vi "init daq state.vi"(0 "Default Setpoint (C)":dbl=30.0, 7 "DAQ state start in":T8 {"T cont"."utility"."therm volt" format="%_6g"; "T cont"."utility"."heat volt in" format="%_6g"; "T cont"."utility"."heat volt out" format="%_6g"; "T cont"."utility"."power out" format="%_6g"; "T cont"."utility"."H Vmax" format="%_6g"; "T cont"."exec"."man power" format="%_6g"; "T cont"."exec"."exec setpoint" format="%_6g"; "T cont"."T params"."Settle Time" step=1.0; "T cont"."T params"."Settle Bandwidth" step=0.01; "T cont"."T params"."Derivative Tme" step=0.01; "T cont"."T params"."Integral Time" step=1.0; "T cont"."T params"."Control Bandwidth" step=0.1; "T cont"."T params"."Setpoint" step=0.1; "T cont"."T status"."Setpoint" format="%_6g"; "T cont"."T status"."Power" format="%_6g"; "T cont"."T status"."Temp" format="%_6g"}, 11 "T cont wait time (ms)":i32=300) -> (4 "T cont out for global update":T1={"exec"={"T mode"=enum."Listening to exec", "exec setpoint"=30.0, "reset"=FALSE, "man power"=0.5, "man"=FALSE, "log"=FALSE, "clear"=FALSE}, "T status"={"Control status"=enum."Below Control Band", "Temp"=0.0, "Power"=0.0, "Time in settle band"=0.0, "Settled"=FALSE, "Low"=FALSE, "High"=FALSE, "Setpoint"=30.0, "Control"=FALSE, "In Settle Band"=FALSE}, "T params"={"Setpoint"=30.0, "Control Bandwidth"=4.0, "Integral Time"=30.0, "Int\nON"=TRUE, "Derivative Tme"=0.5, "Der\nON"=TRUE, "Settle Bandwidth"=1.0, "Settle Time"=60.0}, "utility"={"meas index"=0, "wait (ms)"=300, "H Vmax"=8.5, "power out"=0.0, "heat volt out"=0.0, "heat volt in"=0.0, "therm volt"=0.0, "t T P hist"=[], "cont hist"=[]}} {"utility"."therm volt" format="%_6g"; "utility"."heat volt in" format="%_6g"; "utility"."heat volt out" format="%_6g"; "utility"."power out" format="%_6g"; "utility"."H Vmax" format="%_6g"; "exec"."man power" format="%_6g"; "exec"."exec setpoint" format="%_6g"; "T params"."Settle Time" step=1.0; "T params"."Settle Bandwidth" step=0.01; "T params"."Derivative Tme" step=0.01; "T params"."Integral Time" step=1.0; "T params"."Control Bandwidth" step=0.1; "T params"."Setpoint" step=0.1; "T status"."Setpoint" format="%_6g"; "T status"."Power" format="%_6g"; "T status"."Temp" format="%_6g"}, 8 "DAQ state start out":T8 {"T cont"."utility"."therm volt" format="%_6g"; "T cont"."utility"."heat volt in" format="%_6g"; "T cont"."utility"."heat volt out" format="%_6g"; "T cont"."utility"."power out" format="%_6g"; "T cont"."utility"."H Vmax" format="%_6g"; "T cont"."exec"."man power" format="%_6g"; "T cont"."exec"."exec setpoint" format="%_6g"; "T cont"."T params"."Settle Time" step=1.0; "T cont"."T params"."Settle Bandwidth" step=0.01; "T cont"."T params"."Derivative Tme" step=0.01; "T cont"."T params"."Integral Time" step=1.0; "T cont"."T params"."Control Bandwidth" step=0.1; "T cont"."T params"."Setpoint" step=0.1; "T cont"."T status"."Setpoint" format="%_6g"; "T cont"."T status"."Power" format="%_6g"; "T cont"."T status"."Temp" format="%_6g"})   [LabVIEW 2019]
doc: "Thus subvi initializes the temp daq state machine and the global variables for the bug experiment.\n\nPaul K Dixon\nP3600\nCSUSB Physics"
uses:
  typedefs/DAQ T state cluster.ctl
  typedefs/DAQ T state enum.ctl
  typedefs/temp cont cluster.ctl
  typedefs/temp exec cluster.ctl
  typedefs/temp mode enum.ctl
  typedefs/temp indicator.ctl
  typedefs/temp control status.ctl
  typedefs/PID control parameters.ctl
  typedefs/temp cont utility.ctl
panel:
  in  "T cont.T status":T4={"Control status"=enum."Below Control Band", "Temp"=25.0, "Power"=0.0, "Time in settle band"=0.0, "Settled"=FALSE, "Low"=TRUE, "High"=FALSE, "Setpoint"=30.0, "Control"=FALSE, "In Settle Band"=FALSE} {"Setpoint" format="%_6g"; "Power" format="%_6g"; "Temp" format="%_6g"}
  in  "T cont.T params":T6={"Setpoint"=30.0, "Control Bandwidth"=4.0, "Integral Time"=20.0, "Int\nON"=TRUE, "Derivative Tme"=0.2, "Der\nON"=TRUE, "Settle Bandwidth"=1.0, "Settle Time"=60.0} {"Settle Time" step=1.0; "Settle Bandwidth" step=0.01; "Derivative Tme" step=0.01; "Integral Time" step=1.0; "Control Bandwidth" step=0.1; "Setpoint" step=0.1}
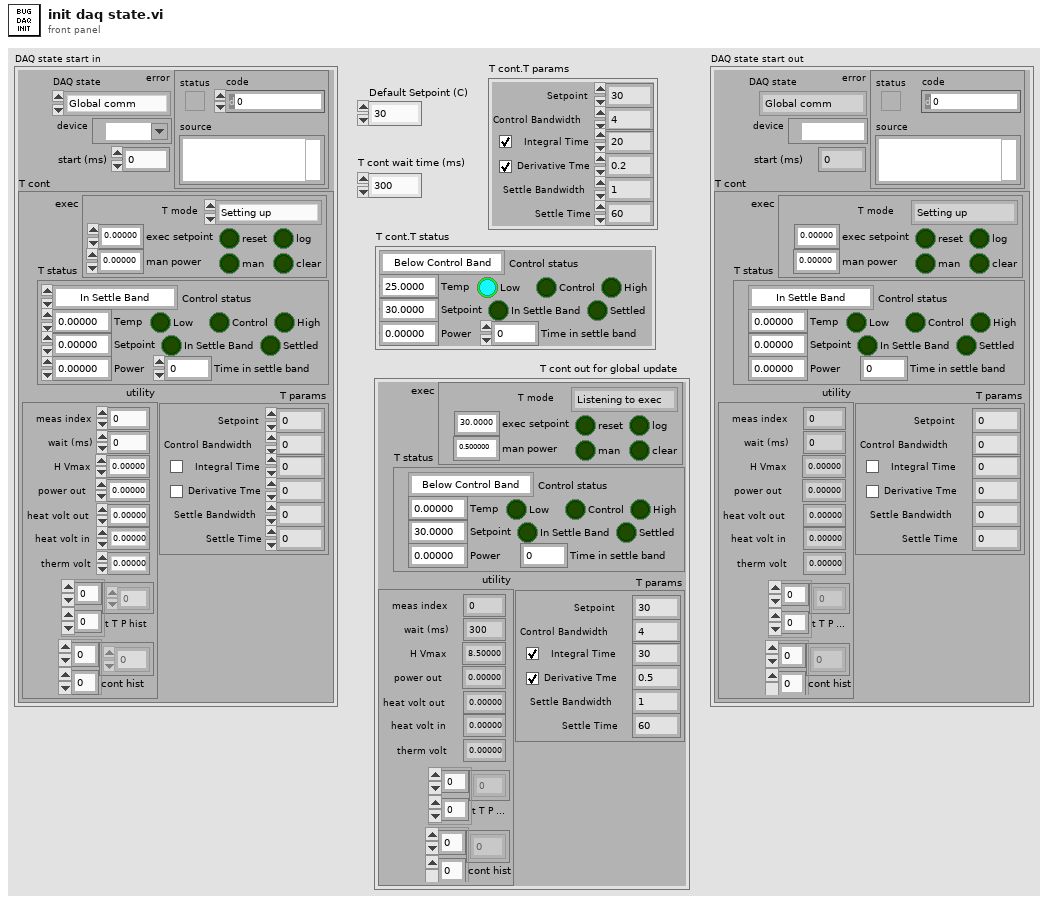
[diagram p1: front panel]
types:
  T1 = typedef "temp cont cluster.ctl" = cluster{"exec":T2, "T status":T4, "T params":T6, "utility":T7}
  T2 = typedef "temp exec cluster.ctl" = cluster{"T mode":T3, "exec setpoint":dbl, "reset":bool, "man power":dbl, "man":bool, "log":bool, "clear":bool}
  T3 = typedef "temp mode enum.ctl" = enum16{"Setting up", "Listening to exec", "Exit"}
  T4 = typedef "temp indicator.ctl" = cluster{"Control status":T5, "Temp":dbl, "Power":dbl, "Time in settle band":dbl, "Settled":bool, "Low":bool, "High":bool, "Setpoint":dbl, "Control":bool, "In Settle Band":bool}
  T5 = typedef "temp control status.ctl" = enum16{"In Settle Band", "In Control Band", "Below Control Band", "Above Control Band"}
  T6 = typedef "PID control parameters.ctl" = cluster{"Setpoint":dbl, "Control Bandwidth":dbl, "Integral Time":dbl, "Int\nON":bool, "Derivative Tme":dbl, "Der\nON":bool, "Settle Bandwidth":dbl, "Settle Time":dbl}
  T7 = typedef "temp cont utility.ctl" = cluster{"meas index":i32, "wait (ms)":i32, "H Vmax":dbl, "power out":dbl, "heat volt out":dbl, "heat volt in":dbl, "therm volt":dbl, "t T P hist":dbl[][], "cont hist":dbl[][]}
  T8 = typedef "DAQ T state cluster.ctl" = cluster{"DAQ state":T9, "device":tag, "start (ms)":i32, "error":errorcluster, "T cont":T1}
  T9 = typedef "DAQ T state enum.ctl" = enum16{"Global comm", "Meas T & P", "PID power calc", "Man Power set", "Output Power", "Wait", "Exit"}
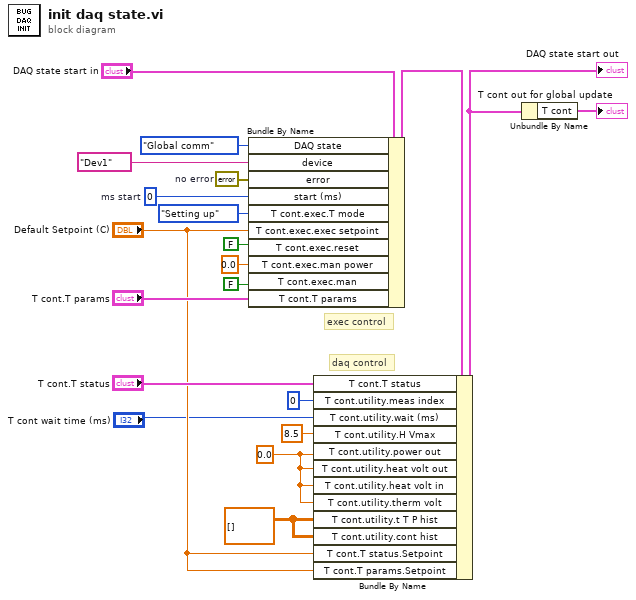
[diagram p0: block diagram]
diagram:
  w4 = 0.0 ("T cont.H Vmax")
  w3 = dbl[][] [] ("T cont.T hist")
  w11 = u32 0  # ms start
  w15 = errorcluster {"status"=FALSE, "code"=0, "source"=""}  # no error
  # "daq control"
  # "exec control"
  n1 = Bundle By Name(cluster="DAQ state start in", "DAQ state"=DAQ_T_state_enum."Global comm", "device"=tag "Dev1", "error"=w15, "start (ms)"=w11, "T cont.exec.T mode"=temp_mode_enum."Setting up", "T cont.exec.exec setpoint"="Default Setpoint (C)", "T cont.exec.reset"=FALSE, "T cont.exec.man power"=0.0, "T cont.exec.man"=FALSE, "T cont.T params"="T cont.T params") -> (w13:T8)
  n2 = Bundle By Name(cluster=w13, "T cont.T status"="T cont.T status", "T cont.utility.meas index"=0 ("T cont.therm volt"), "T cont.utility.wait (ms)"="T cont wait time (ms)", "T cont.utility.H Vmax"=8.5 ("T cont.H Vmax"), "T cont.utility.power out"=w4, "T cont.utility.heat volt out"=w4, "T cont.utility.heat volt in"=w4, "T cont.utility.therm volt"=w4, "T cont.utility.t T P hist"=w3, "T cont.utility.cont hist"=w3, "T cont.T status.Setpoint"="Default Setpoint (C)", "T cont.T params.Setpoint"="Default Setpoint (C)") -> (w2:T8)
  "DAQ state start out" <- w2
  n3 = Unbundle By Name(w2) -> ("T cont"=→"T cont out for global update":T1)
